vi "kvCanIoCtlSetTxReqs.vi"(2 "error in (no error)":errorcluster, 3 "Transmit Requests":enum16{"Off", "On"}(ring), 4 "Channel Handle (input only)":i32) -> (0 "error out":errorcluster, 1 "Channel Handle (ouput only)":i32)   [LabVIEW 2022 SP3]
doc: "Set Transmit Requests off or on. Off is the default."
uses:
  canlib32.dll
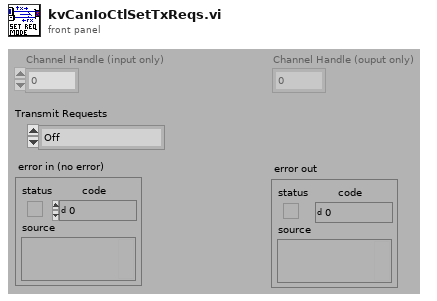
[diagram p1: front panel]
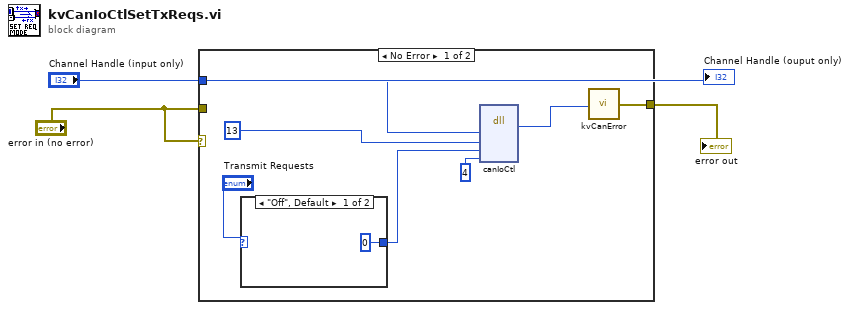
[diagram p0: block diagram]
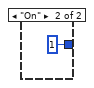
[diagram p2: hidden frame]
diagram:
  n1 = case shown="No Error" "error in (no error)" {
    tunnel: [w10 w13] -> w3
    tunnel: "error in (no error)" -> [_ w13]
    tunnel: "Channel Handle (input only)" -> [w8 _]
    frame No Error {
      n2 = case shown="\"Off\", Default" "Transmit Requests" {
        tunnel: [0 1] -> w4
        frame "Off", Default {
        }
        frame "On" {
        }
      }
      n3 = dll-call lib="canlib32.dll" fn="canIoCtl" label="Call canIoCtl"("handle"=w8, "func"=13, "buf"=w4, "buflen"=4) -> (w9:i32)  [unwired: 7 in, 2 out]
      n4 = call "kvCanError.vi"("error code"=w9) -> ("error out"=w10:errorcluster)
    }
    frame Error {
    }
  }
  "error out" <- w3
  "Channel Handle (ouput only)" <- "Channel Handle (input only)"
